vi "LabView.vi"() -> ()   [LabVIEW 2023]
uses:
  <vilib>/MakerHub/LINX/Public/Peripherals/Digital/Digital Write 1 Chan.vi
  <vilib>/MakerHub/LINX/Public/Peripherals/Digital/Digital Write N Chans.vi
  <vilib>/MakerHub/LINX/Private/Local IO/LinxDigitalWrite.vi
  <vilib>/MakerHub/LINX/Public/Utilities/Check Channel.vi
  <vilib>/MakerHub/LINX/Public/Utilities/Open Serial.vi
  <vilib>/MakerHub/LINX/Private/Utilties/Generate Error.vi
  <vilib>/MakerHub/LINX/LMH-LINX.lvlib
  <vilib>/httpClient/LabVIEWHTTPClient.lvlib
panel:
  in  "Field":i8
  out "String":string
  in  "FieldValue":dbl
  in  "API Key":string
  in  "Stop":bool
  in  "LED_OnOff":bool
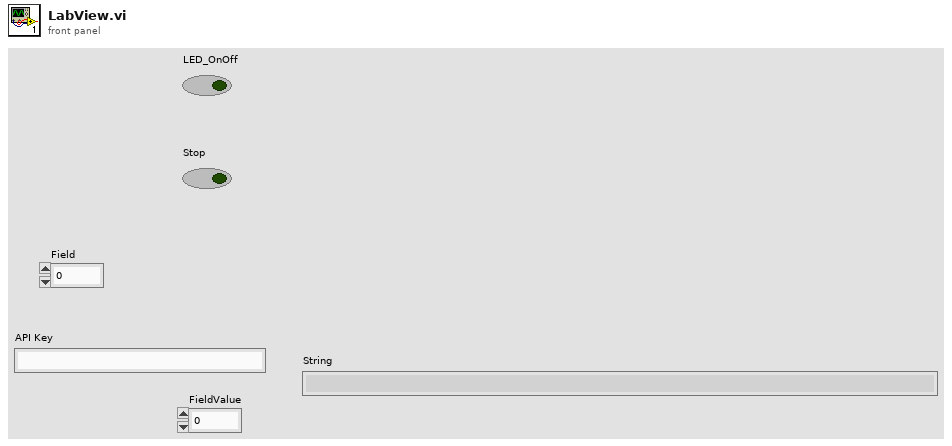
[diagram p1: front panel]
types:
  T1 = typedef "LabVIEWHTTPClient.lvlib/ClientHandle.ctl" = refnum<k1>
  T2 = typedef "LMH-LINX.lvlib/LINX Ref.ctl" = cluster{"IO":T3, "Interface":T4, "LINX Device Config":T5}
  T3 = typedef "LMH-LINX.lvlib/Platform.ctl" = enum16{"Remote", "Local"}
  T4 = typedef "LMH-LINX.lvlib/Interface.ctl" = enum16{"Serial", "TCP"}
  T5 = typedef "LMH-LINX.lvlib/Device.lvlib/LINX Device Config.ctl" = cluster{"Interface":T4, "COM Port":refnum<visa-resource-name>, "TCP Configuration":T6, "Device Family":u8, "Device ID":u8, "Device Name":string, "TCP Ref":refnum<k5>, "Channels":T7}
  T6 = typedef "LMH-LINX.lvlib/Device.lvlib/TCP Config.ctl" = cluster{"IP Address":string, "Port":u16}
  T7 = typedef "LMH-LINX.lvlib/Channels.ctl" = cluster{"DI":u8[], "DO":u8[], "AI":u8[], "AO":u8[], "PWM":u8[], "QE":u8[], "UART":u8[], "I2C 2":u8[], "SPI":u8[], "CAN":u8[], "Servo":u8[], "AI Ref (V)":dbl, "AI Resolution (Bits)":u8, "AO Ref (V)":dbl, "AO Resolution (Bits)":u8}
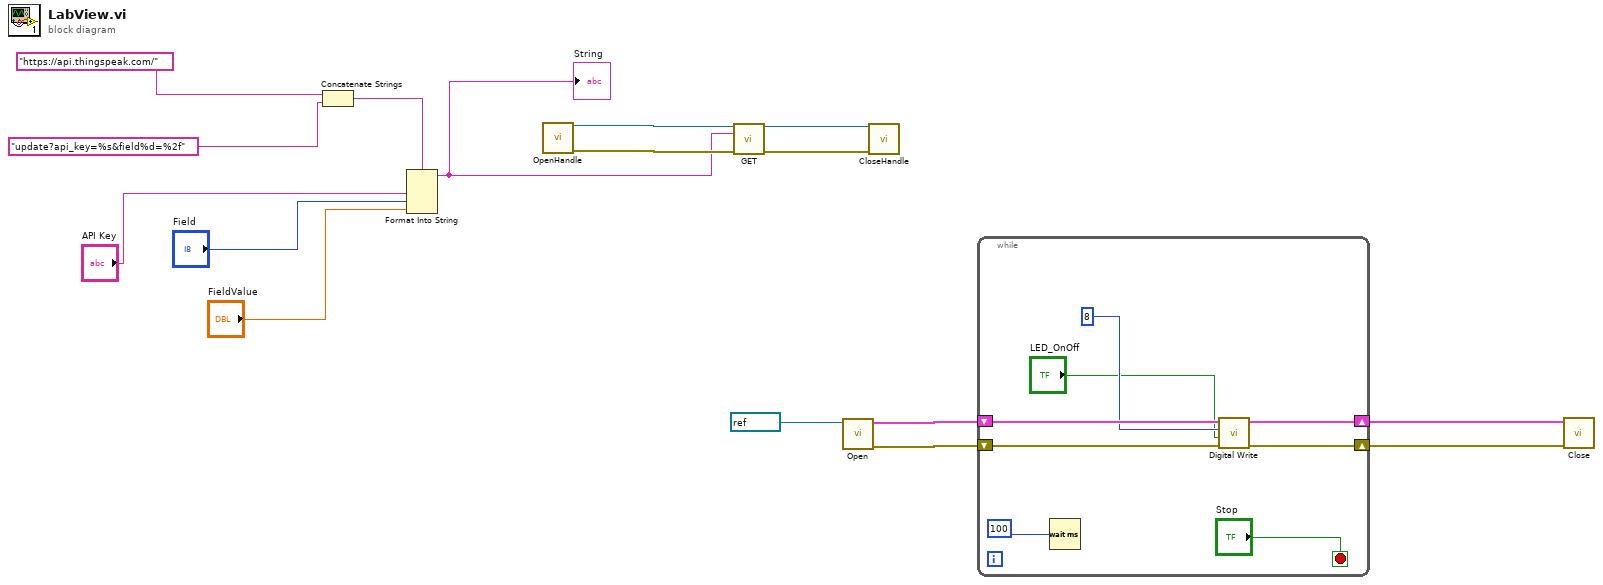
[diagram p0: block diagram]
diagram:
  n1 = Concatenate Strings("https://api.thingspeak.com/", "update?api_key=%s&field%d=%2f") -> (w1:string)
  n2 = Format Into String(format string=w1, "API Key", "Field", "FieldValue") -> (resulting string=w3:string)  [unwired: 2 in, 1 out]
  "String" <- w3
  n3 = call <vilib>:"OpenHandle.vi"() -> ("client handle out"=w9:T1, "error out"=w8:errorcluster)  [unwired: 14 in]
  n4 = call <vilib>:"GET.vi"("client handle"=w9, "url"=w3, "error in (no error)"=w8) -> ("client handle out"=w10:T1, "error out"=w11:errorcluster)  [unwired: 9 in, 2 out]
  n5 = call-poly <vilib>:"Open.vi"("Serial Port"=refnum<visa-resource-name> "N/A") -> ("Error Out"=w15:errorcluster, "LINX Resource"=w14:T2)  [unwired: 8 in, 1 out]
  n6 = call <vilib>:"CloseHandle.vi"("client handle"=w10, "error in (no error)"=w11) -> ()  [unwired: 13 in, 1 out]
  n7 = while {
    shift-right: [w21] -> w12
    shift-left: w15 -> [w24]
    shift-right: [w22] -> w13
    shift-left: w14 -> [w23]
    stop <- "Stop" stop-if-true
    n8 = Wait (ms)(milliseconds to wait=u32 100) -> ()  [unwired: 1 out]
    n9 = call-poly <vilib>:"Digital Write.vi"("Error In"=w24, "Output Value"="LED_OnOff", "DO Channel"=u8 8, "LINX Resource"=w23) -> ("Error Out"=w21:errorcluster, "LINX Resource"=w22:T2)  [unwired: 6 in]
  }
  n10 = call <vilib>:"Close.vi"("Error In"=w12, "LINX Resource"=w13) -> ()  [unwired: 9 in, 1 out]
